vi "check if variants are equal.vi"(8 "error in (no error)":errorcluster, 9 "Variant in":variant, 10 "Variant in":variant, 11 "Dynamic Cluster Test in":refnum<class "Variant Data Manipulation Tests.lvclass">) -> (0 "error out":errorcluster, 3 "Dynamic Cluster Test out":refnum<class "Variant Data Manipulation Tests.lvclass">)   [LabVIEW 2017, in "Variant Data Manipulation Tests.lvclass"]
uses:
  Variant Data Manipulation Tests.lvclass
  Source/Variant Data Manipulation.lvlib
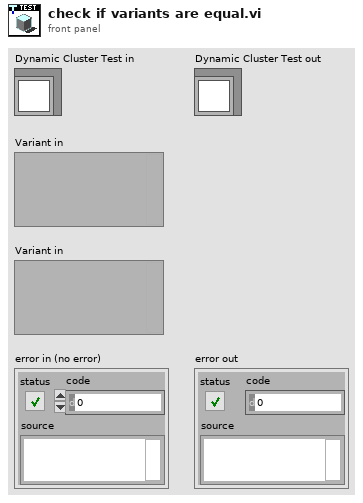
[diagram p1: front panel]
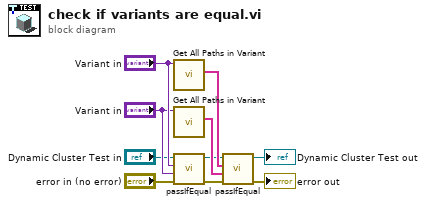
[diagram p0: block diagram]
diagram:
  n1 = call "Get All Paths in Variant.vi"("Variant in"="Variant in") -> ("Paths out"=w7:string[])  [unwired: 8 in, 2 out]
  n2 = call "Get All Paths in Variant.vi"("Variant in"="Variant in") -> ("Paths out"=w9:string[])  [unwired: 8 in, 2 out]
  n3 = call-dynamic "passIfEqual.vi"("error in (no error)"="error in (no error)", "y"="Variant in", "x"="Variant in", "TestCase in"="Dynamic Cluster Test in") -> ("error out"=w2:errorcluster, "TestCase out"=w5:refnum<class "Variant Data Manipulation Tests.lvclass">)  [unwired: 6 in]
  n4 = call-dynamic "passIfEqual.vi"("error in (no error)"=w2, "y"=w9, "x"=w7, "TestCase in"=w5) -> ("error out"=→"error out":errorcluster, "TestCase out"=→"Dynamic Cluster Test out":refnum<class "Variant Data Manipulation Tests.lvclass">)  [unwired: 6 in]
